vi "ExcelWritev2.vi"(8 "error in":errorcluster, 10 "Data":string[][](array[string])) -> (0 "error out":errorcluster)   [LabVIEW 2015]
uses:
  <vilib>/Utility/NIReport.llb/Append Text Table to Report (wrap).vi
  <vilib>/Utility/NIReport.llb/NI_report.lvclass
  SR430 Driver VIs/SR430Driver.lvlib
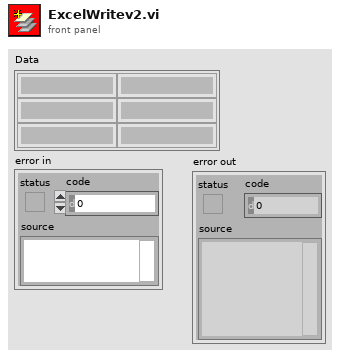
[diagram p1: front panel]
types:
  T1 = enum16{"Standard Report", "HTML", "Word", "Excel"}
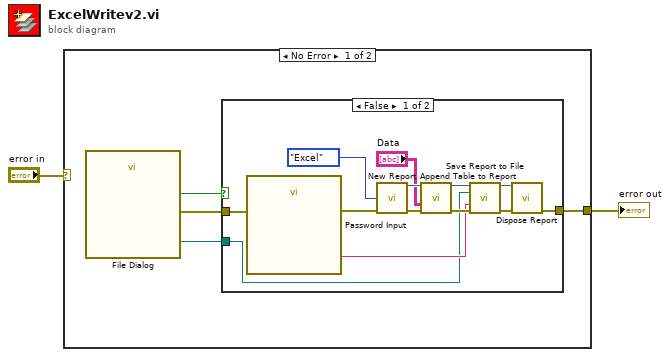
[diagram p0: block diagram]
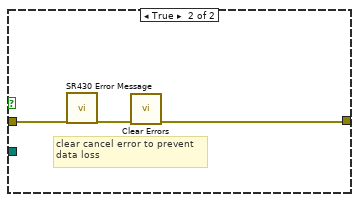
[diagram p2: hidden frame]
diagram:
  n1 = case shown="No Error" "error in" {
    selector: "error in" -> [_ w23]
    tunnel: [w5 w23] -> w2
    frame No Error {
      n2 = call "File Dialog"() -> ("selected path"=w4:path, "cancelled"=w3:bool, "error out"=w6:errorcluster)  [unwired: 12 in, 1 out]
      n3 = case shown="False" w3 {
        tunnel: w6 -> [w9 w22]
        tunnel: [w8 w20] -> w5
        tunnel: w4 -> [w7 _]
        frame False {
          n4 = call "Password Input"("error in (no error)"=w9) -> ("Password"=w11:string, "error out"=w10:errorcluster)  [unwired: 16 in, 1 out]
          n5 = call <vilib>:"New Report.vi"("report type"=T1."Excel", "error in (no error)"=w10) -> ("report out"=w19:refnum<class "NI_report.lvclass">, "error out"=w18:errorcluster)  [unwired: 12 in]
          n6 = call-poly <vilib>:"Append Table to Report.vi"("report in"=w19, "text data"="Data", "error in (no error)"=w18) -> ("report out"=w17:refnum<class "NI_report.lvclass">, "error out"=w16:errorcluster)  [unwired: 9 in, 2 out]
          n7 = call-dynamic "Save Report to File.vi"("report in"=w17, "report file path"=w7, "password (\"\")"=w11, "error in (no error)"=w16) -> ("report out"=w15:refnum<class "NI_report.lvclass">, "error out"=w14:errorcluster)  [unwired: 10 in]
          n8 = call-dynamic "Dispose Report.vi"("report in"=w15, "error in (no error)"=w14) -> ("error out"=w8:errorcluster)  [unwired: 13 in]
        }
        frame True {
          # "clear cancel error to prevent \ndata loss"
          n9 = call "SR430 Error Message.vi"("error in (no error)"=w22) -> ("error out"=w21:errorcluster)  [unwired: 15 in, 3 out]
          n10 = call <vilib>:"Clear Errors.vi"("error in (no error)"=w21) -> ("error out"=w20:errorcluster)  [unwired: 5 in, 1 out]
        }
      }
    }
    frame Error {
    }
  }
  "error out" <- w2
